vi "FGV - AO.vi"(8 "error in":errorcluster, 10 "Digital Outs":dbl[](array[numeric])=[0.0, 0.0], 11 "State":T1) -> (0 "error out":errorcluster)   [LabVIEW 2017]
doc: "v1.1:\n- 2WR motor selection\n\nv1.0:\n- VI Created"
uses:
  controls/FGV AO.ctl
  <vilib>/DAQmx/write.llb/DAQmx Write (Analog 1D DBL NChan 1Samp).vi
  <vilib>/DAQmx/miscellaneous.llb/DAQmx Fill In Error Info.vi
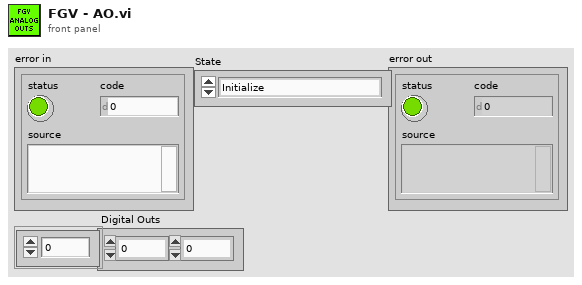
[diagram p1: front panel]
types:
  T1 = typedef "FGV AO.ctl" = enum16{"Initialize", "Write AO", "Clear Tasks"}
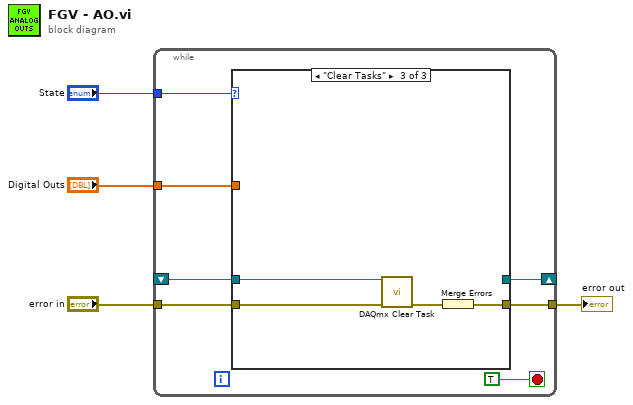
[diagram p0: block diagram]
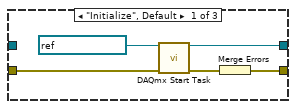
[diagram p2: hidden frame]
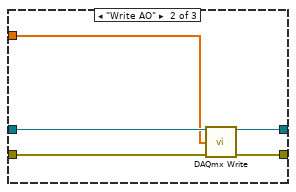
[diagram p3: hidden frame]
diagram:
  n1 = while {
    tunnel: "State" -> [w11]
    shift-right: [w10] -> _
    shift-left: _ -> [w7]
    tunnel: "error in" -> [w8]
    tunnel: [w9] -> w2
    tunnel: "Digital Outs" -> [w6]
    stop <- TRUE stop-if-true
    n2 = case shown="\"Clear Tasks\"" w11 {
      tunnel: [w16 w18 _] -> w10
      tunnel: [w15 w20 w25] -> w9
      tunnel: w8 -> [w14 w21 w22]
      tunnel: w7 -> [_ w19 w24]
      tunnel: w6 -> [_ w17 _]
      frame "Initialize", Default {
        n3 = call <vilib>:"DAQmx Start Task.vi"("task/channels in"=refnum<k21> "1903_AllAO", "error in"=w14) -> ("task out"=w16:refnum<k21>, "error out"=w12:errorcluster)  [unwired: 12 in]
        n4 = Merge Errors(w12) -> (w15:errorcluster)
      }
      frame "Write AO" {
        n5 = call-poly <vilib>:"DAQmx Write.vi"("task/channels in"=w19, "data"=w17, "error in"=w21) -> ("task out"=w18:refnum<k21>, "error out"=w20:errorcluster)  [unwired: 10 in, 1 out]
      }
      frame "Clear Tasks" {
        n6 = call <vilib>:"DAQmx Clear Task.vi"("task in"=w24, "error in"=w22) -> ("error out"=w23:errorcluster)  [unwired: 13 in]
        n7 = Merge Errors(w23) -> (w25:errorcluster)
      }
    }
  }
  "error out" <- w2
